vi "Simple NATS Client Publisher.vi"() -> ()   [LabVIEW 2024]
uses:
  VIs/NATS PUB.vi
  VIs/subVIs/Set Timeout.vi
  VIs/subVIs/Validate CONNECT.vi
  VIs/NATS PING.vi
  <vilib>/Utility/error.llb/Trim Whitespace.vi
  <vilib>/dlg_ctls.llb/Space Constant.vi
  VIs/subVIs/Check for Authorization.vi
  VIs/subVIs/Add Version and Language JSON Entries.vi
  <vilib>/Utility/error.llb/Trim Whitespace One-Sided.vi
  VIs/subVIs/Package Version Constant.vi
  VIs/NATS READ.vi
  NATS Core.lvlib
panel:
  in  "subject":string="TestSubject"
  in  "timeout ms (5000)":i32=5000
  in  "port (4222)":u16=4222
  in  "NATS server address":string="localhost"
  out "error out":errorcluster
  in  "stop":bool
  # "Set prior to execution"
  # "Visit https://nats.io to download the free, open-source NATS server"
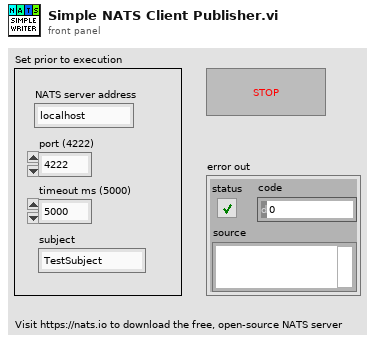
[diagram p1: front panel]
types:
  T1 = typedef "NATS Core.lvlib/nats connection.ctl" = cluster{"connection ID":refnum<k5>, "server INFO":string, "timeout ms":i32, "verbose?":bool, "server headers?":bool, "client headers?":bool}
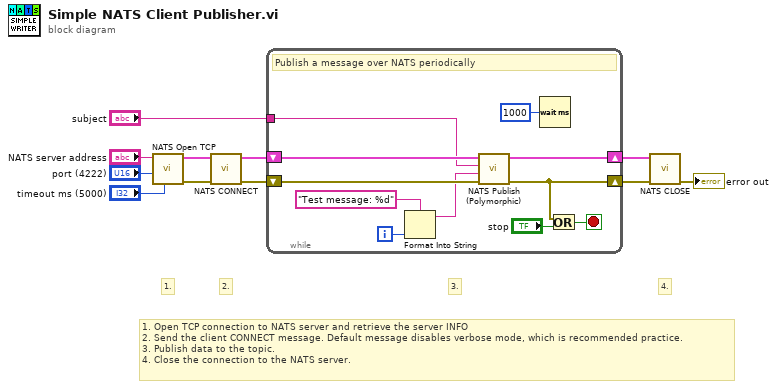
[diagram p0: block diagram]
diagram:
  # "1. Open TCP connection to NATS server and retrieve the server INFO\n2. Send the client CONNECT message. Default message disables verbose mode, which is recommended practice.\n3. Publish data to the topic.\n4. Close the connection to the NATS server."
  # "4."
  # "3."
  # "2."
  # "1."
  n1 = call "NATS Open TCP.vi"("timeout ms (5000)"="timeout ms (5000)", "port (4222)"="port (4222)", "address"="NATS server address") -> ("error out"=w9:errorcluster, "nats connection"=w11:T1)  [unwired: 5 in, 2 out]
  n2 = call "NATS CONNECT.vi"("error in"=w9, "nats connection in"=w11) -> ("error out"=w8:errorcluster, "nats connection out"=w10:T1)  [unwired: 7 in, 1 out]
  n3 = while {
    shift-right: [w20] -> w7
    shift-left: w10 -> [w21]
    shift-right: [w18] -> w6
    shift-left: w8 -> [w19]
    tunnel: "subject" -> [w16]
    i -> [w14]
    stop <- w17 stop-if-true
    # "Publish a message over NATS periodically"
    n4 = Format Into String(format string="Test message: %d", w14) -> (resulting string=w13:string)  [unwired: 2 in, 1 out]
    n5 = call-poly "NATS Publish (Polymorphic).vi"("error in"=w19, "payload"=w13, "subject"=w16, "nats connection in"=w21) -> ("error out"=w18:errorcluster, "dup nats connection"=w20:T1)  [unwired: 6 in]
    n6 = Wait (ms)(milliseconds to wait=u32 1000) -> ()  [unwired: 1 out]
    n7 = Or(x=w18, y="stop") -> (x .or. y?=w17:bool)
  }
  n8 = call "NATS CLOSE.vi"("error in"=w6, "nats connection in"=w7) -> ("error out"=→"error out":errorcluster)  [unwired: 9 in]
